vi "Read N Circles Progress.vi"(8 "Error In":errorcluster, 11 "Leap Handle":T1) -> (0 "Error Out":errorcluster, 2 "All Circle Progress":dbl[](array[numeric]), 3 "Leap Handle":T1)   [LabVIEW 2011, in "LVH-Leap.lvlib"]
doc: "Read N circle gestures progresss."
uses:
  LVH-Leap.lvlib
  Private/Type Defs/Leap Handle.ctl
  C:/github/labviewhacker/LVH-Leap/LabVIEW/vi.lib/LabVIEW Hacker/Leap/Private/Libs/LeapCSharp.NET3.5.dll
  Private/Libs/LeapCSharp.NET3.5.dll
  Read N Circles.vi
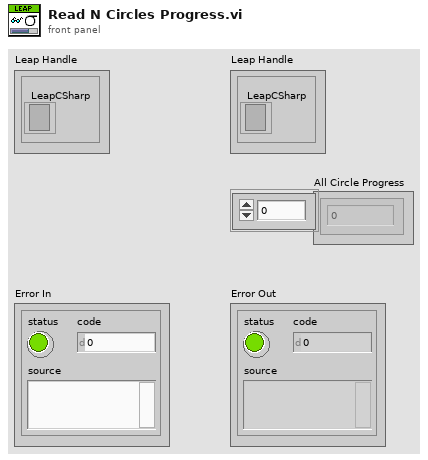
[diagram p1: front panel]
types:
  T1 = typedef "LVH-Leap.lvlib/Leap Handle.ctl" = cluster{"LeapCSharp":refnum<k24>}
  T2 = typedef "LVH-Leap.lvlib/Gesture Circle.ctl" = cluster{"Common":T3, "Center":T6, "Normal":T6, "Progress":dbl, "Radius":dbl}
  T3 = typedef "LVH-Leap.lvlib/Gesture Common.ctl" = cluster{"ID":dbl, "Duration (S)":dbl, "Gesture Type":T4, "Gesture State":T5}
  T4 = typedef "LVH-Leap.lvlib/Gesture Type.ctl" = enum16{"Invalid", "Swipe", "Circle", "Screen Tap", "Key Tap"}
  T5 = typedef "LVH-Leap.lvlib/Gesture State.ctl" = enum16{"Invalid", "Start", "Update", "Stop"}
  T6 = typedef "LVH-Leap.lvlib/Vector.ctl" = cluster{"Pitch":sgl, "Yaw":sgl, "Roll":sgl, "Magnitude":sgl, "XYZ":sgl[]}
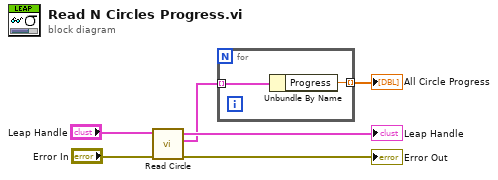
[diagram p0: block diagram]
diagram:
  n1 = call-poly "Read Circle.vi"("Error In"="Error In", "Leap Handle"="Leap Handle") -> ("Error Out"=→"Error Out":errorcluster, "All Circles Data"=w2:T2[], "Leap Handle"=→"Leap Handle":T1)  [unwired: 6 in, 1 out]
  n2 = for {
    tunnel: [w8] -> w1 mode=indexing
    tunnel: w2 -> [w7] mode=indexing
    n3 = Unbundle By Name(w7) -> ("Progress"=w8:dbl)
  }
  "All Circle Progress" <- w1
